vi "LabView360-6-Global.vi"() -> ()   [LabVIEW 2017]
panel:
  in  "停止":bool
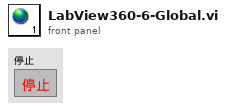
[diagram p1: front panel]
diagram:
